vi "SET_LayerType.vi"(8 "error in (no error)":errorcluster, 10 "Type":T1, 11 "Layer.lvclass in":refnum<class "Layer.lvclass">) -> (0 "error out":errorcluster, 3 "Layer.lvclass out":refnum<class "Layer.lvclass">)   [LabVIEW 2020, in "Layer.lvclass"]
doc: "Specify the User Layer Type."
uses:
  <vilib>/LabVIEW Icon API/lv_icon/Classes/Layer/Layer.lvclass
  <vilib>/LabVIEW Icon API/lv_icon/Controls/LayerType.ctl
  <vilib>/LabVIEW Icon API/lv_icon/Classes/Layer/Layer.lvclass/Layer.ctl
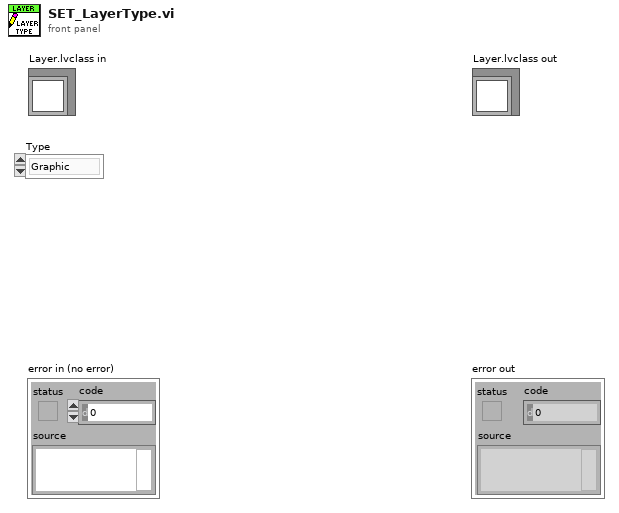
[diagram p1: front panel]
types:
  T1 = typedef "LayerType.ctl" = enum16{"Graphic", "Text", "Tool", "Graphic Drop"}
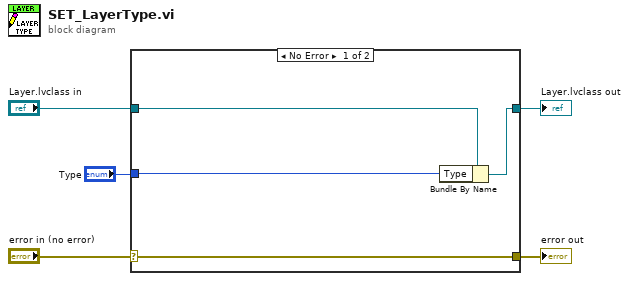
[diagram p0: block diagram]
diagram:
  n1 = case shown="No Error" "error in (no error)" {
    selector: "error in (no error)" -> [w9 w10]
    tunnel: [w9 w10] -> w4
    tunnel: [w7 w11] -> w2
    tunnel: "Layer.lvclass in" -> [w8 w11]
    tunnel: "Type" -> [w6 _]
    frame No Error {
      n2 = Bundle By Name(cluster=w8, "Type"=w6) -> (w7:refnum<class "Layer.lvclass">)
    }
    frame Error {
    }
  }
  "error out" <- w4
  "Layer.lvclass out" <- w2
